vi "Finding Angle Protections.vi"(0 "Distance 1":dbl format="%0.2f", 1 "Distance 2":dbl format="%0.2f") -> (2 "Trigger?":bool, 3 "Angle to Turn":dbl, 4 "Current Angle":dbl)   [LabVIEW 2019]
uses:
  <vilib>/ptbypt/NI_PtbyPt.lvlib
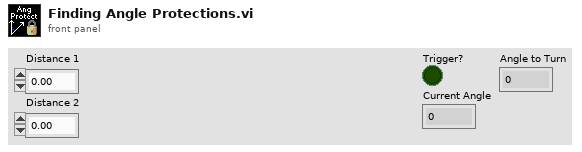
[diagram p1: front panel]
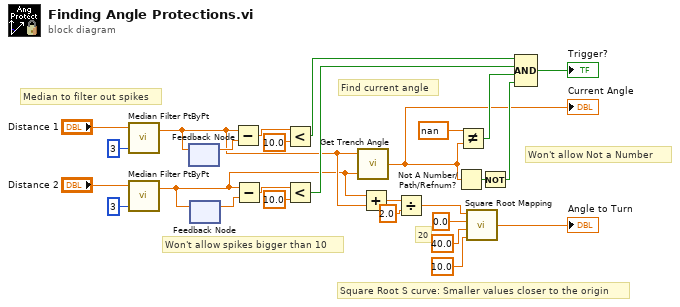
[diagram p0: block diagram]
diagram:
  # "Won't allow Not a Number"
  # "Square Root S curve: Smaller values closer to the origin"
  # "Find current angle"
  # "Won't allow spikes bigger than 10"
  # "Median to filter out spikes"
  # "20"
  n1 = call <vilib>:"Median Filter PtByPt.vi"("rank"=3, "x"="Distance 1") -> ("Filtered x"=w8:dbl)  [unwired: 2 in, 1 out]
  n2 = call <vilib>:"Median Filter PtByPt.vi"("rank"=3, "x"="Distance 2") -> ("Filtered x"=w6:dbl)  [unwired: 2 in, 1 out]
  n3 = feedback #1() -> (w24:dbl)  [unwired: 1 in]
  n4 = feedback-in #1(w8) -> ()
  n5 = feedback #2() -> (w23:dbl)  [unwired: 1 in]
  n6 = feedback-in #2(w6) -> ()
  n7 = Subtract(x=w8, y=w24) -> (x-y=w20:dbl)
  n8 = Subtract(x=w6, y=w23) -> (x-y=w17:dbl)
  n9 = Less?(x=w20, y=10.0) -> (x < y?=w22:bool)
  n10 = Less?(x=w17, y=10.0) -> (x < y?=w18:bool)
  n11 = call "Get Trench Angle.vi"("Distance 2"=w6, "Distance 1"=w8) -> ("Current Angle"=w5:dbl)  [unwired: 1 in]
  "Current Angle" <- w5
  n12 = Add(x=w6, y=w8) -> (x+y=w27:dbl)
  n13 = Divide(x=w27, y=2.0) -> (x/y=w16:dbl)
  n14 = Not A Number/Path/Refnum?(number/path/refnum=w5) -> (NaN/Path/Refnum?=w13:bool)
  n15 = Not Equal?(x=nan, y=w5) -> (x != y?=w25:bool)
  n16 = call "Square Root Mapping.vi"("x"=w16, "Min Distance"=0.0 ("Min A"), "Max Distance"=40.0 ("Max A"), "Angle"=10.0 ("Max B")) -> ("Angle to Turn"=→"Angle to Turn":dbl)  [unwired: 4 in]
  n17 = Not(x=w13) -> (.not. x?=w12:bool)
  n18 = Compound Arithmetic op=AND(w22, w18, w25, w12) -> (→"Trigger?":bool)
